vi "Test Heart Rate calc (FFT method).vi"() -> ()   [LabVIEW 2015]
panel:
  out "Waveform Graph":dbl[](graph)
  in  "Path":path=path "D:/Data/TTH DATA/ekg-1.f64"
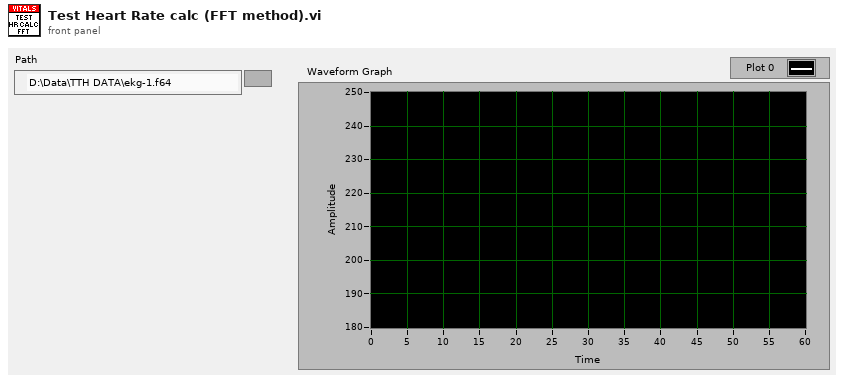
[diagram p1: front panel]
types:
  T1 = typedef "DL-File Header.ctl" = cluster{"path":path, "nchan":i32, "names":string[], "Fs (Hz)":dbl, "pts/read/ch":i32, "header size":i32, "nrecords":i32, "last read":i32, "bytes/read":i32}
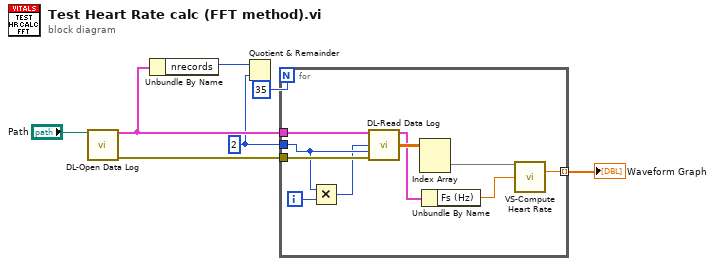
[diagram p0: block diagram]
diagram:
  w2 = 2
  n1 = call "DL-Open Data Log.vi"("Path"="Path") -> ("Header"=w4:T1, "error out"=w6:errorcluster)  [unwired: 13 in]
  n2 = Unbundle By Name(w4) -> ("nrecords"=w3:i32)
  n3 = Quotient & Remainder(x=w3, y=w2) -> ()  [unwired: 2 out]
  n4 = for {
    N: 35 -> [_]
    tunnel: w4 -> [w17]
    tunnel: w6 -> [w16]
    tunnel: [w11] -> w5 mode=indexing
    tunnel: w2 -> [w9]
    i -> [w10]
    n5 = Multiply(x=w9, y=w10) -> (x*y=w8:i32)
    n6 = call "DL-Read Data Log.vi"("Header in"=w17, "First"=w8, "N"=w9, "error in (no error)"=w16) -> ("Header out"=w14:T1, "Array"=w15:dbl[][])  [unwired: 9 in, 1 out]
    n7 = Index Array(array=w15) -> (element=w13:dbl[])  [unwired: 2 in]
    n8 = Unbundle By Name(w14) -> ("Fs (Hz)"=w12:dbl)
    n9 = call "VS-Compute Heart Rate.vi"("ECG"=w13, "Sampling Rate (Hz)"=w12) -> ("Heart Rate (bpm)"=w11:dbl)  [unwired: 11 in, 2 out]
  }
  "Waveform Graph" <- w5
